vi "gps_speed_estimation_with_fb.vi"(8 "Maximum Window":i32=5, 9 "Longitude":dbl, 10 "Latitude":dbl) -> (3 "GPS":T1)   [LabVIEW 2023]
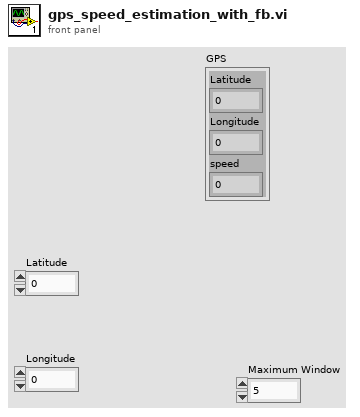
[diagram p1: front panel]
types:
  T1 = cluster{"Latitude":dbl, "Longitude":dbl, "speed":dbl}
  T2 = cluster{"Latitude":dbl, "Longitude":dbl, "Filtered x":dbl}
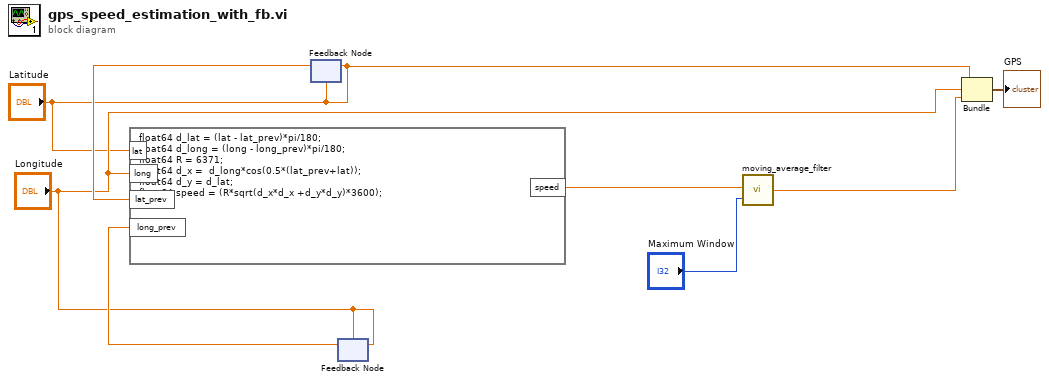
[diagram p0: block diagram]
diagram:
  n1 = feedback #1("Latitude") -> (w6:dbl)
  n2 = feedback-in #1("Latitude") -> ()
  n3 = feedback #2("Longitude") -> (w7:dbl)
  n4 = formula code="float64 d_lat = (lat - lat_prev)*pi/180;\nfloat64 d_long = (long - long_prev)*pi/180;\nfloat64 R = 6371;\nfloat64 d_x =  d_long*cos(0.5*(lat_prev+lat));\nfloat64 d_y = d_lat;\nfloat64 speed = (R*sqrt(d_x*d_x +d_y*d_y)*3600);"("lat"="Latitude", "lat_prev"=w6, "long"="Longitude", "long_prev"=w7) -> ("speed"=w2:dbl)
  n5 = feedback-in #2("Longitude") -> ()
  n6 = call "moving_average_filter.vi"("Maximum Window"="Maximum Window", "X"=w2) -> ("Filtered x"=w3:dbl)
  n7 = Bundle("Latitude"="Latitude", "Longitude"="Longitude", "Filtered x"=w3) -> (→"GPS":T2)  [unwired: 1 in]
